vi "_WSAStartup.vi"(8 "Error In":errorcluster) -> (0 "Error out":errorcluster, 3 "&wsaData":u8[](array[numeric]) format="%02x")   [LabVIEW 2018]
uses:
  ws2_32.dll
panel:
  out "szSystemStatus":string
  out "wHighVersion":dbl
  out "wVersion":dbl
  out "szDescription":string
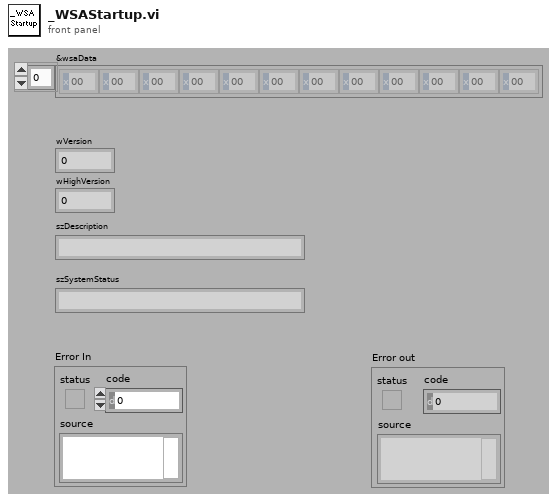
[diagram p1: front panel]
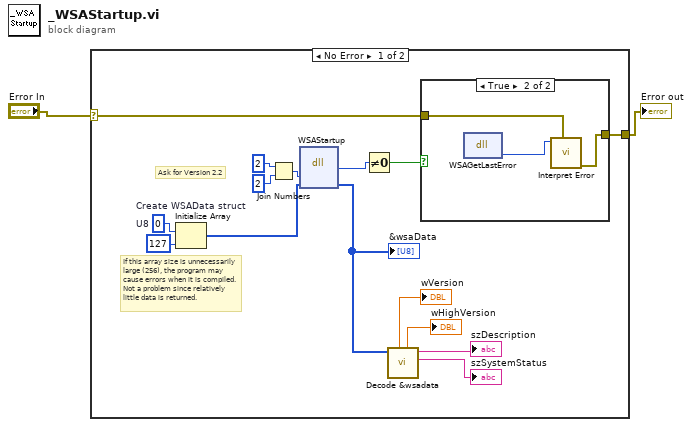
[diagram p0: block diagram]
diagram:
  n1 = case shown="No Error" "Error In" {
    selector: "Error In" -> [w10 w22]
    tunnel: [w9 w22] -> w1
    frame No Error {
      w13 = u8 0  # U8
      # "If this array size is unnecessarily\nlarge (256), the program may \ncause errors when it is compiled.\nNot a problem since relatively\nlittle data is returned."
      # "Ask for Version 2.2"
      n2 = Initialize Array "Create WSAData struct"(w13, 127) -> (w12:u8[])
      n3 = Join Numbers(hi=u8 2, lo=u8 2) -> ((hi.lo)=w17:u16)
      n4 = dll-call lib="ws2_32.dll" fn="WSAStartup"("Version"=w17, "&wsaData"=w12) -> (w8:i32, "&wsaData"=w7:u8[])  [unwired: 4 in, 2 out]
      "&wsaData" <- w7
      n5 = Not Equal To 0?(x=w8) -> (x != 0?=w11:bool)
      n6 = call "Decode &wsadata.vi"("&wsdata"=w7) -> ("szSystemStatus"=→"szSystemStatus":string, "szDescription"=→"szDescription":string, "wHighVersion"=→"wHighVersion":dbl, "wVersion"=→"wVersion":dbl)  [unwired: 5 in, 2 out]
      n7 = case shown="True" w11 {
        tunnel: w10 -> [w18 w21]
        tunnel: [w18 w20] -> w9
        frame False {
        }
        frame True {
          n8 = dll-call lib="ws2_32.dll" fn="WSAGetLastError"() -> (w19:i32)  [unwired: 3 in, 2 out]
          n9 = call "Interpret Error.vi"("Error In"=w21, "Code"=w19) -> ("Error Out"=w20:errorcluster)  [unwired: 9 in]
        }
      }
    }
    frame Error {
    }
  }
  "Error out" <- w1
